vi "debug VI.vi"(5 "x output":dbl[](array[numeric]), 7 "x input":dbl[](array[numeric]), 8 "error in (no error)":errorcluster, 10 "Output":dbl[](array[numeric]), 11 "input array":dbl[](array[numeric])) -> ()   [LabVIEW 2011, in "Interpolate 1D Array Custom Device.lvlib"]
uses:
  Interpolate 1D Array Custom Device.lvlib
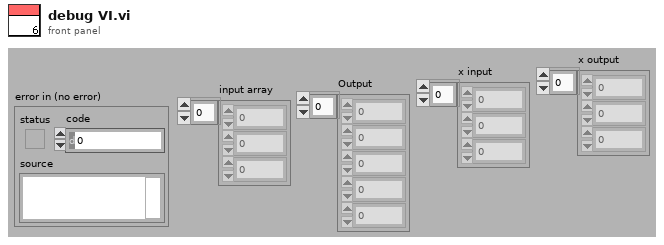
[diagram p1: front panel]
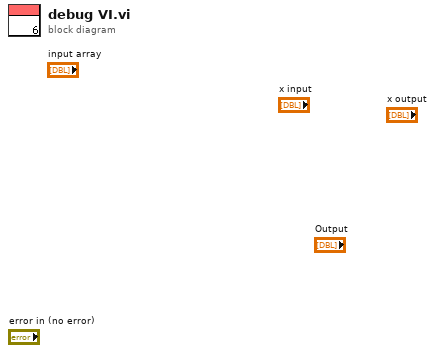
[diagram p0: block diagram]
diagram:
